vi "字符串处理.vi"(11 "输入字符串":string) -> (3 "输出字符串":string)   [LabVIEW 2020]
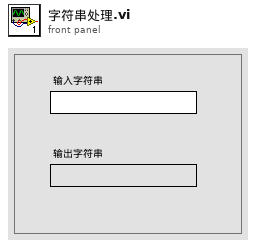
[diagram p1: front panel]
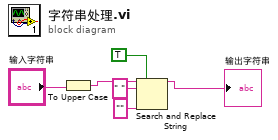
[diagram p0: block diagram]
diagram:
  n1 = To Upper Case(1:"输入字符串") -> (0:w5:string)
  n2 = Search and Replace String(replace all?=TRUE ("替换全部？(F)"), input string=w5, search string=" " ("搜索字符串"), replace string="" ("替换字符串(\"\")")) -> (result string=→"输出字符串":string)  [unwired: 4 in, 3 out]
